vi "GV-ConvRangeGraph.vi"(10 "RangeL":dbl, 11 "RangeH":dbl) -> (2 "Offset":dbl, 3 "Gain":dbl)   [LabVIEW 2020, in "Gviewer.lvclass"]
doc: "Convert RangeH and RangeL into Gain and Offset for Graph display"
uses:
  Gviewer.lvclass
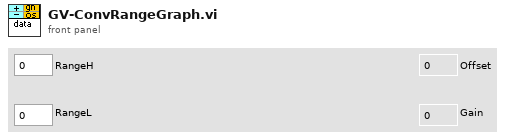
[diagram p1: front panel]
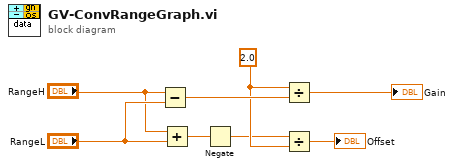
[diagram p0: block diagram]
diagram:
  w3 = 2.0 ("x")
  n1 = Subtract(x="RangeH", y="RangeL") -> (x-y=w8:dbl)
  n2 = Add(x="RangeH", y="RangeL") -> (x+y=w4:dbl)
  n3 = Negate(x=w4) -> (-x=w2:dbl)
  n4 = Divide(x=w3, y=w8) -> (x/y=→"Gain":dbl)
  n5 = Divide(x=w2, y=w3) -> (x/y=→"Offset":dbl)
